vi "Cull and GroupPegPYLB.vi"(6 "Line Border":cluster{"Top":dbl, "Bottom":dbl}={"Top"=6.0, "Bottom"=1.0}, 9 "Score Cutoff":dbl=3.0, 10 "Sorted Data":dbl[][](array[numeric])) -> (0 "Rect":T1, 1 "Line":T1, 2 "Score":dbl, 3 "Center":cluster{"X":dbl, "Y":dbl})   [LabVIEW 2016]
doc: "Examine the particle measurements to find the most likely pair that make up the target. This mostly compares the edges of the bounding boxes. It then returns information about the overall target, notably the rectangle sourrounding the particles, the vertical line that bisects the target, and the center of the top particle."
panel:
  out "Grouping Scores":T2(array[cluster])
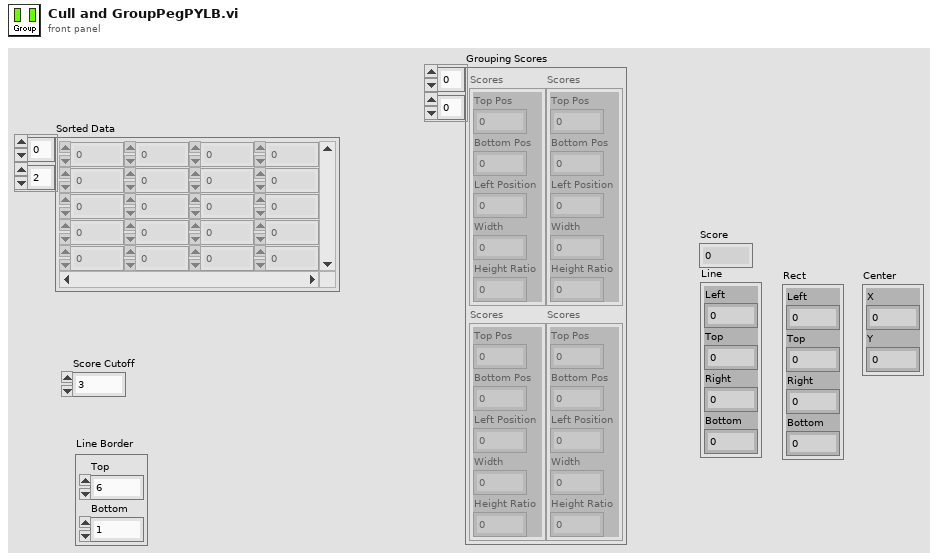
[diagram p1: front panel]
types:
  T1 = cluster{"Left":dbl, "Top":dbl, "Right":dbl, "Bottom":dbl}
  T2 = cluster{"Top Pos":dbl, "Bottom Pos":dbl, "Left Position":dbl, "Width":dbl, "Height Ratio":dbl}[][]
  T3 = cluster{"Top Position":dbl, "Bottom Position":dbl, "Left Gap":dbl, "Width":dbl, "Height Ratio":dbl}
  T4 = cluster{"Left":dbl, "Numeric":dbl, "Right":dbl, "Numeric":dbl}
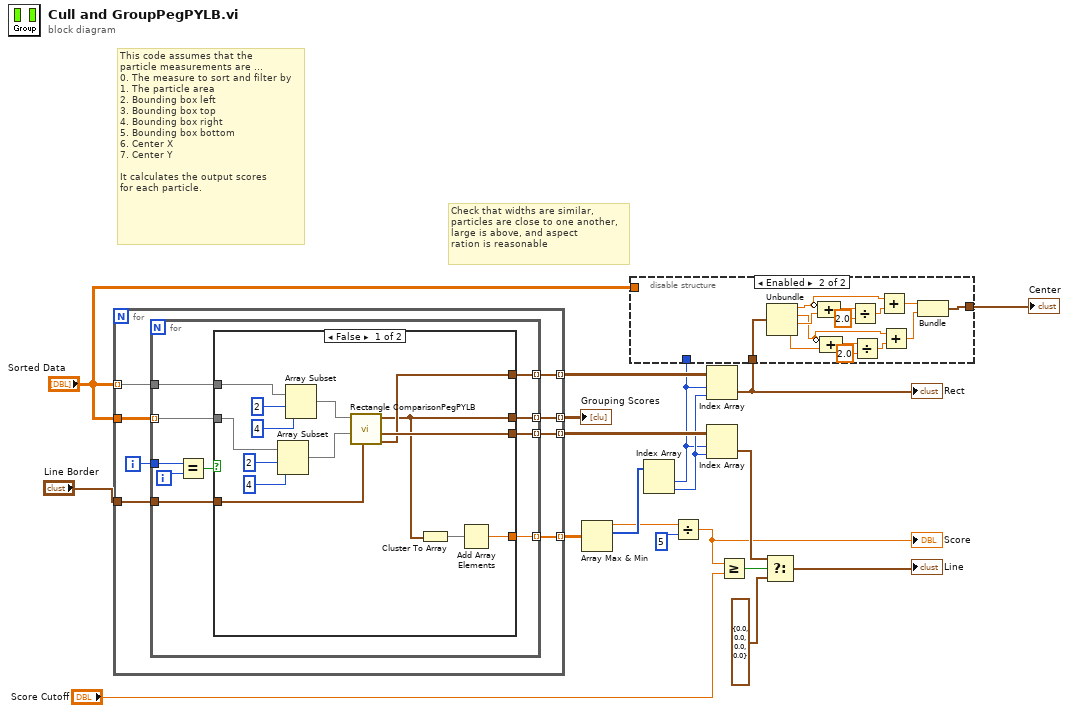
[diagram p0: block diagram]
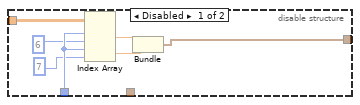
[diagram p2: hidden frame]
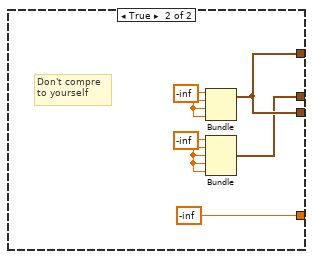
[diagram p3: hidden frame]
diagram:
  # "Check that widths are similar,\nparticles are close to one another,\nlarge is above, and aspect\nration is reasonable"
  # "This code assumes that the\nparticle measurements are ...\n0. The measure to sort and filter by\n1. The particle area\n2. Bounding box left\n3. Bounding box top\n4. Bounding box right\n5. Bounding box bottom\n6. Center X\n7. Center Y\n\nIt calculates the output scores\nfor each particle."
  n1 = for {
    tunnel: "Sorted Data" -> [w27] mode=indexing
    tunnel: "Sorted Data" -> [w26]
    tunnel: [w25] -> w19 mode=indexing
    tunnel: [w23] -> w18 mode=indexing
    tunnel: [w22] -> w15 mode=indexing
    tunnel: [w21] -> w11 mode=indexing
    tunnel: "Line Border" -> [w20]
    i -> [w24]
    n2 = for {
      tunnel: w27 -> [w37]
      tunnel: w26 -> [w35] mode=indexing
      tunnel: [w34] -> w25 mode=indexing
      tunnel: w24 -> [w33]
      tunnel: [w31] -> w23 mode=indexing
      tunnel: [w30] -> w22 mode=indexing
      tunnel: [w29] -> w21 mode=indexing
      tunnel: w20 -> [w28]
      i -> [w32]
      n3 = Equal?(x=w33, y=w32) -> (x = y?=w36:bool)
      n4 = case shown="False" w36 {
        tunnel: w37 -> [w49 _]
        tunnel: w35 -> [w46 _]
        tunnel: [w39 w52] -> w34
        tunnel: [w44 -inf] -> w31
        tunnel: [w41 w55] -> w30
        tunnel: [w40 w55] -> w29
        tunnel: w28 -> [w38 _]
        frame False {
          n5 = Array Subset(array=w46, index=2, length=4) -> (w42:dbl[])
          n6 = Array Subset(array=w49, index=2, length=4) -> (w43:dbl[])
          n7 = call "Rectangle ComparisonPegPYLB.vi"("Line Border"=w38, "Second"=w42, "First"=w43) -> ("Rect"=w40:T1, "Line"=w41:T1, "Scores"=w39:T3)  [unwired: 6 in]
          n8 = Cluster To Array(cluster=w39) -> (array=w45:dbl[])
          n9 = Add Array Elements(numeric array=w45) -> (sum=w44:dbl)
        }
        frame True {
          w53 = -inf
          w54 = -inf
          # "Don't compre\nto yourself"
          n10 = Bundle(w54, w54, w54, w54) -> (w55:cluster{dbl, dbl, dbl, dbl})  [unwired: 1 in]
          n11 = Bundle(w53, w53, w53, w53, w53) -> (w52:cluster{dbl, dbl, dbl, dbl, dbl})  [unwired: 1 in]
        }
      }
    }
  }
  "Grouping Scores" <- w19
  n12 = Array Max & Min(array=w18) -> (max value=w5:dbl, max index (indices)=w6:i32[])  [unwired: 2 out]
  n13 = Index Array(array=w6) -> (element #1=w8:i32, element #2=w10:i32)  [unwired: 2 in]
  n14 = Divide(x=w5, y=5 ("length")) -> (x/y=w4:dbl)
  "Score" <- w4
  n15 = Index Array(array=w11, index (row)=w8, index (col)=w10) -> (element=w1:T1)
  "Rect" <- w1
  n16 = disable-structure shown="Enabled" {
    disable-tunnel: "Sorted Data" -> [w63 _]
    disable-tunnel: w8 -> [w62 _]
    disable-tunnel: [w58 w77] -> w7
    disable-tunnel: w1 -> [_ w76]
    frame Disabled {
      n17 = Index Array(array=w63, index (row) #1=w62, index (col) #1=6 ("index"), index (row) #2=w62, index (col) #2=7 ("index")) -> (element #1=w60:dbl, element #2=w59:dbl)
      n18 = Bundle("Numeric"=w60, "Numeric"=w59) -> (w58:cluster{"Numeric":dbl, "Numeric":dbl})  [unwired: 1 in]
    }
    frame Enabled {
      n19 = Unbundle(w76) -> ("Left"=w71:dbl, "Top"=w65:dbl, "Right"=w75:dbl, "Bottom"=w66:dbl)
      n20 = Compound Arithmetic op=ADD(invert w71, w75) -> (w74:dbl)
      n21 = Compound Arithmetic op=ADD(invert w65, w66) -> (w67:dbl)
      n22 = Divide(x=w74, y=2.0) -> (x/y=w72:dbl)
      n23 = Divide(x=w67, y=2.0) -> (x/y=w69:dbl)
      n24 = Add(x=w71, y=w72) -> (x+y=w70:dbl)
      n25 = Add(x=w65, y=w69) -> (x+y=w64:dbl)
      n26 = Bundle(w70, w64) -> (w77:cluster{dbl, dbl})  [unwired: 1 in]
    }
  }
  "Center" <- w7
  n27 = Index Array(array=w15, index (row)=w8, index (col)=w10) -> (element=w14:T1)
  n28 = Greater Or Equal?(x=w4, y="Score Cutoff") -> (x >= y?=w17:bool)
  n29 = Select(t=w14, s=w17, f=cluster{dbl, "Numeric":dbl, dbl, "Numeric":dbl} {0.0, "Numeric"=0.0, 0.0, "Numeric"=0.0}) -> (s? t:f=→"Line":T4)
